vi "Get State by Index.vi"(8 "error in (no error)":errorcluster, 10 "index":i32, 11 "Example App Properties in":refnum<class "Example App Properties.lvclass">) -> (0 "error out":errorcluster, 2 "Enum":T1, 3 "Example App Properties out":refnum<class "Example App Properties.lvclass">)   [LabVIEW 2015, in "Example Application.lvlib" / "Example App Properties.lvclass"]
uses:
  Example App Properties.lvclass
  DUT State -- Enum.ctl
  Example App Properties.lvclass/Example App Properties.ctl
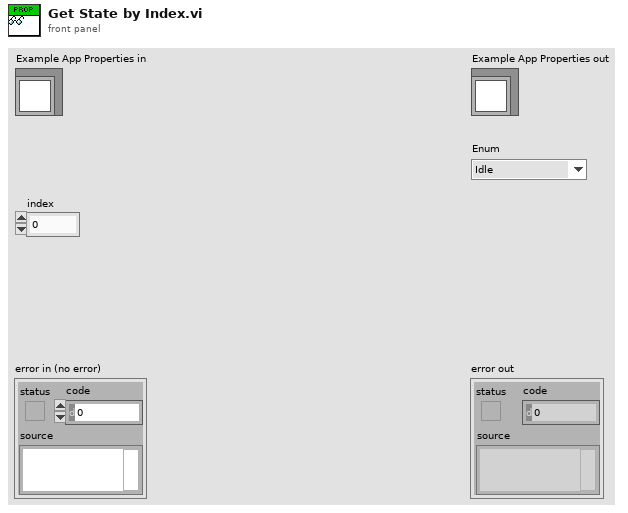
[diagram p1: front panel]
types:
  T1 = typedef "Example Application.lvlib/Example App Properties.lvclass/DUT State -- Enum.ctl" = enum16{"Idle", "Testing", "Passed", "Failed"}
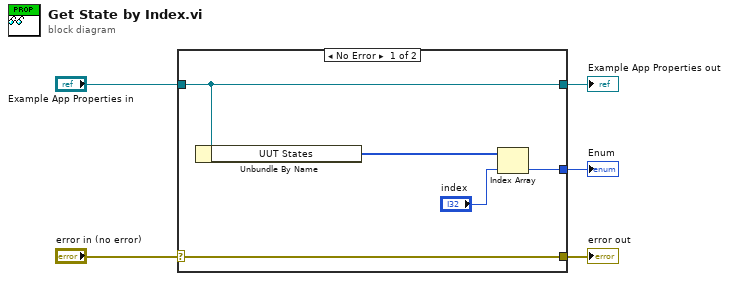
[diagram p0: block diagram]
diagram:
  n1 = case shown="No Error" "error in (no error)" {
    selector: "error in (no error)" -> [w10 w11]
    tunnel: [w10 w11] -> w4
    tunnel: [w9 w12] -> w2
    tunnel: "Example App Properties in" -> [w9 w12]
    tunnel: [w6 _] -> w1
    frame No Error {
      n2 = Unbundle By Name(w9) -> ("UUT States"=w8:T1[])
      n3 = Index Array(array=w8, index="index") -> (element=w6:T1)
    }
    frame Error {
    }
  }
  "error out" <- w4
  "Example App Properties out" <- w2
  "Enum" <- w1
